vi "Path Is Filled.vi"(9 "error in (no error)":errorcluster, 11 "Path in":refnum<class "Path.lvclass">) -> (1 "error out":errorcluster, 2 "x != y?":bool, 3 "Path out":refnum<class "Path.lvclass">)   [LabVIEW 2019, in "Tool Object.lvclass"]
uses:
  Tool Object.lvclass
  Parse/ParsePaths/Path.lvclass
  Parse/ParsePaths/Path.lvclass/Path.ctl
  Parse/CSSProperties/CSSProperties.lvclass/CSSProperties.ctl
  Parse/CSSProperties/CSSProperties.lvclass
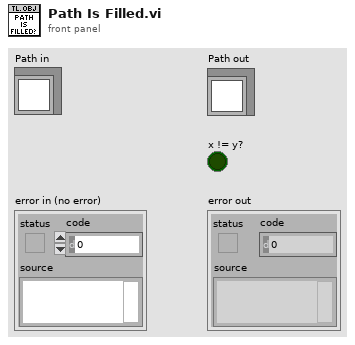
[diagram p1: front panel]
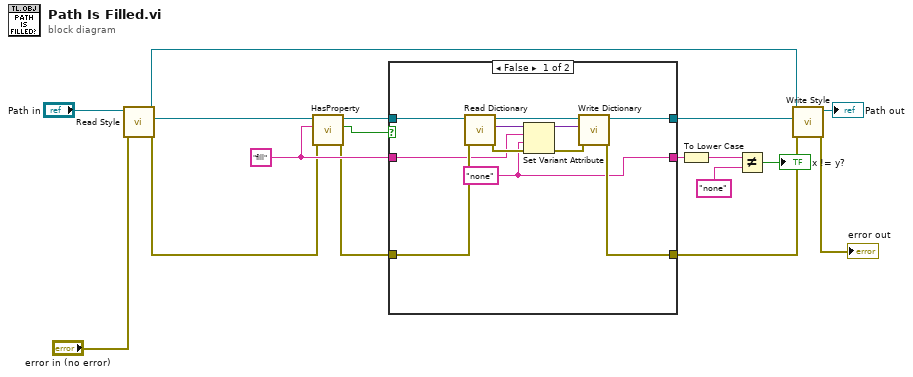
[diagram p0: block diagram]
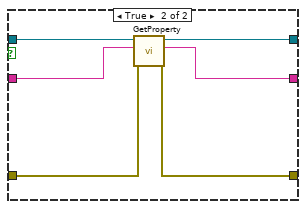
[diagram p2: hidden frame]
diagram:
  w16 = "fill" ("Property")
  n1 = call "Read Style.vi"("error in (no error)"="error in (no error)", "Path in"="Path in") -> ("error out"=w9:errorcluster, "CSSProperties.lvclass"=w11:refnum<class "CSSProperties.lvclass">, "Path out"=w6:refnum<class "Path.lvclass">)  [unwired: 7 in]
  n2 = call "HasProperty.vi"("error in (no error)"=w9, "Property"=w16, "CSSProperties in"=w11) -> ("error out"=w10:errorcluster, "Exists?"=w17:bool, "CSSProperties out"=w15:refnum<class "CSSProperties.lvclass">)  [unwired: 6 in]
  n3 = case shown="False" w17 {
    tunnel: [w25 w34] -> w8
    tunnel: [w18 w30] -> w14
    tunnel: w15 -> [w24 w33]
    tunnel: w16 -> [w19 w29]
    tunnel: [w23 w32] -> w7
    tunnel: w10 -> [w22 w31]
    frame False {
      w18 = "none" ("Value")
      n4 = call "Read Dictionary.vi"("error in (no error)"=w22, "CSSProperties in"=w24) -> ("error out"=w20:errorcluster, "Dictionary"=w27:variant, "CSSProperties out"=w26:refnum<class "CSSProperties.lvclass">)  [unwired: 7 in]
      n5 = Set Variant Attribute(Variant=w27, name=w19, value=w18, error in=w20) -> (Variant out=w28:variant, error out=w21:errorcluster)  [unwired: 1 out]
      n6 = call "Write Dictionary.vi"("error in (no error)"=w21, "Dictionary"=w28, "CSSProperties in"=w26) -> ("error out"=w23:errorcluster, "CSSProperties out"=w25:refnum<class "CSSProperties.lvclass">)  [unwired: 7 in]
    }
    frame True {
      n7 = call "GetProperty.vi"("error in (no error)"=w31, "Property"=w29, "CSSProperties in"=w33) -> ("error out"=w32:errorcluster, "Value"=w30:string, "CSSProperties out"=w34:refnum<class "CSSProperties.lvclass">)  [unwired: 6 in]
    }
  }
  n8 = To Lower Case(string=w14) -> (all lower case string=w13:string)
  n9 = Not Equal?(x=w13, y="none") -> (x != y?=→"x != y?":bool)
  n10 = call "Write Style.vi"("error in (no error)"=w7, "CSSProperties.lvclass"=w8, "Path in"=w6) -> ("error out"=→"error out":errorcluster, "Path out"=→"Path out":refnum<class "Path.lvclass">)  [unwired: 7 in]
